vi "CRYUnflatten Results.vi"(11 "Unflatten Result":string) -> (0 "Error?":bool, 2 "Result":T2={"Name"="Test for Signal [L]", "Margin"=nan, "unit"="", "Verdict"=FALSE, "Limit"="", "Max/Min"="", "protected"=FALSE, "Step No."=0, "Test Info"="", "AutoProtect"=FALSE} {"Margin" format="%.2f"}, 3 "Header info":T1={"Data type"="Data            ", "Version"=1, "Dimensions"=0})   [LabVIEW 2013]
uses:
  Typedef Control/CRYResult Cluster.ctl
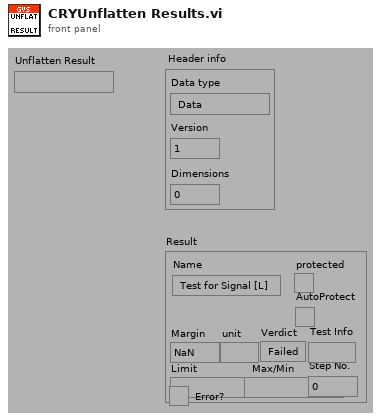
[diagram p1: front panel]
types:
  T1 = cluster{"Data type":string, "Version":u16, "Dimensions":u8}
  T2 = typedef "CRYResult Cluster.ctl" = cluster{"Name":string, "Margin":dbl, "unit":string, "Verdict":bool, "Limit":string, "Max/Min":string, "protected":bool, "Step No.":i32, "Test Info":string, "AutoProtect":bool}
  T3 = cluster{"Name":string, "Margin":dbl, "unit":string, "Verdict":bool, "Limit":string, "Max/Min":string, "protected":bool, "Step No.":i32, "Test Info":string, "AutoProtect":bool}
  T4 = cluster{"unsigned byte array[0]":u8, "unsigned byte array[1]":u8, "unsigned byte array[2]":u8}
  T5 = cluster{"substring":string, u16, "unsigned byte array[2]":u8}
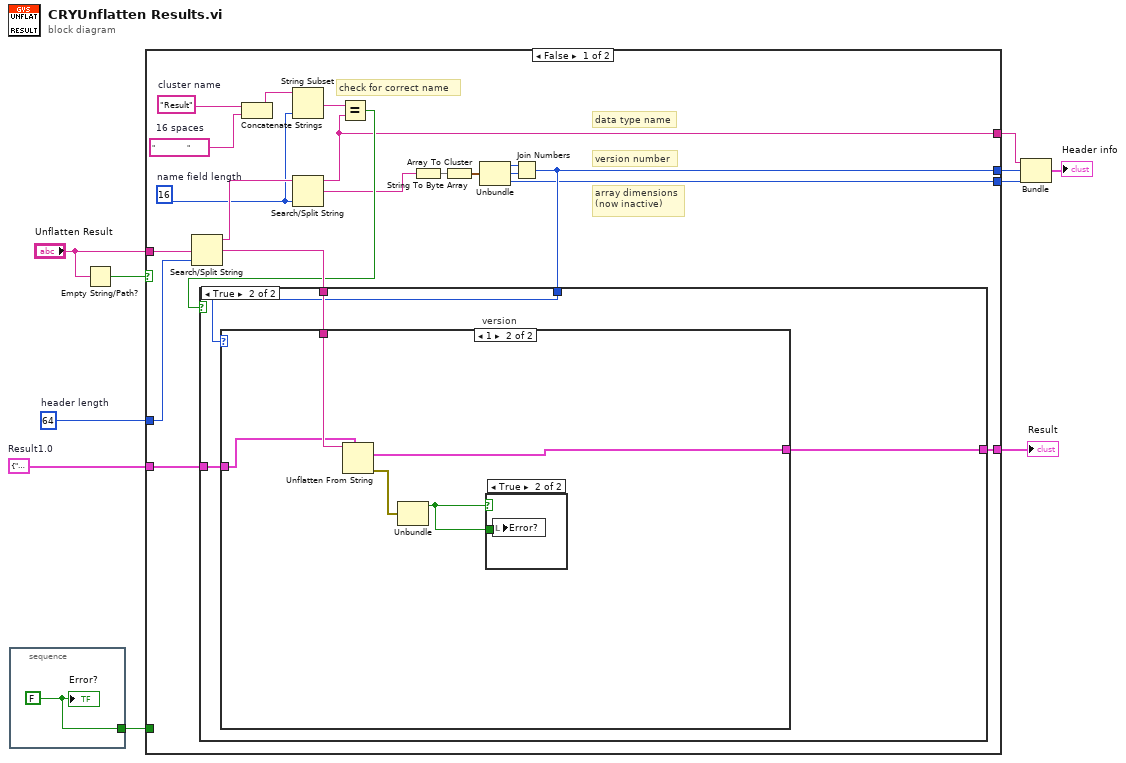
[diagram p0: block diagram]
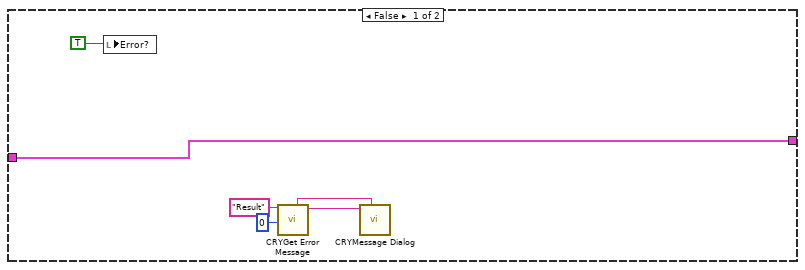
[diagram p2: hidden frame]
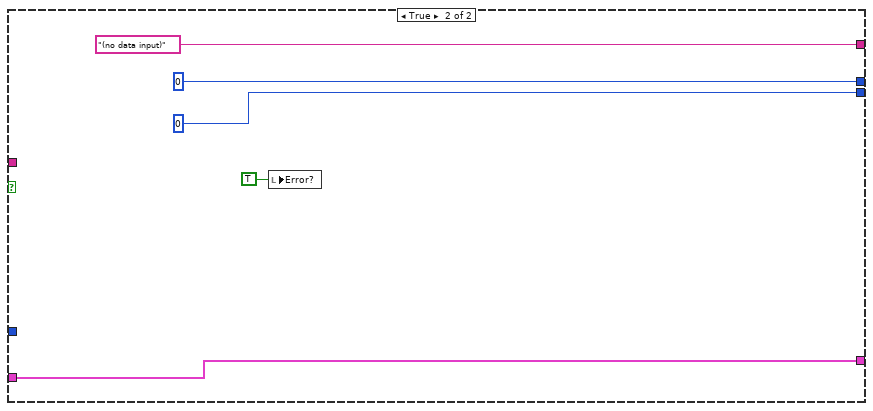
[diagram p5: hidden frame]
diagram:
  w2 = T3 {"Name"="Test for Signal [L]", "Margin"=nan, "unit"="", "Verdict"=FALSE, "Limit"="", "Max/Min"="", "protected"=FALSE, "Step No."=0, "Test Info"="", "AutoProtect"=FALSE}  # Result1.0
  w8 = 64  # header length
  n1 = stacked-sequence {
    tunnel: [w11] -> w3
    frame #0 {
      w11 = FALSE
      "Error?" <- w11
    }
  }
  n2 = Empty String/Path?(string/path="Unflatten Result") -> (empty?=w9:bool)
  n3 = case shown="False" w9 {
    tunnel: "Unflatten Result" -> [w31 _]
    tunnel: w8 -> [w25 _]
    tunnel: [w22 u16 0] -> w6
    tunnel: [w14 u8 0] -> w7
    tunnel: [w15 "(no data input)" ("substring")] -> w5
    tunnel: w3 -> [_ _]
    tunnel: [w13 w49] -> w1
    tunnel: w2 -> [w12 w49]
    frame False {
      w19 = "                "  # 16 spaces
      w20 = "Result"  # cluster name
      w17 = 16  # name field length
      # "check for correct name"
      # "array dimensions\n(now inactive)"
      # "version number"
      # "data type name"
      n4 = Search/Split String(string=w31, offset (0)=w25) -> (substring before match=w24:string, match + rest of string=w26:string)  [unwired: 2 out]
      n5 = Concatenate Strings(w20, w19) -> (w18:string)
      n6 = String Subset(string=w18, length (rest)=w17) -> (substring=w16:string)  [unwired: 1 out]
      n7 = Search/Split String(string=w24, offset (0)=w17) -> (substring before match=w15:string, match + rest of string=w21:string)  [unwired: 2 out]
      n8 = Equal?(x=w16, y=w15) -> (x = y?=w23:bool)
      n9 = String To Byte Array(string=w21) -> (unsigned byte array=w30:u8[])
      n10 = Array To Cluster(array=w30) -> (cluster=w29:T4)
      n11 = Unbundle(w29) -> ("unsigned byte array[0]"=w28:u8, "unsigned byte array[1]"=w27:u8, "unsigned byte array[2]"=w14:u8)
      n12 = Join Numbers(hi=w28, lo=w27) -> ((hi.lo)=w22:u16)
      n13 = case shown="True" w23 {
        tunnel: w26 -> [_ w41]
        tunnel: w22 -> [_ w40]
        tunnel: [w36 w39] -> w13
        tunnel: w12 -> [w36 w38]
        frame False {
          n14 = local write "Error?"(TRUE) -> ()
          n15 = call "CRYGet Error Message.vi"("Error No"=0 ("No"), "Kind"="Result") -> ("Message"=w33:string, "Window Title"=w32:string)  [unwired: 4 in, 4 out]
          n16 = call "CRYMessage Dialog.vi"("Window Title"=w32, "Message Content"=w33) -> ()  [unwired: 8 in, 2 out]
        }
        frame True {
          n17 = case "version" shown="1" w40 {
            tunnel: w41 -> [_ w47]
            tunnel: [w42 w44] -> w39
            tunnel: w38 -> [w42 w45]
            frame Default {
            }
            frame 1 {
              n18 = Unflatten From String(type=w45, binary string=w47) -> (value=w44:T3, error out=w43:errorcluster)  [unwired: 1 in, 3 out]
              n19 = Unbundle(w43) -> ("status"=w46:bool)  [unwired: 2 out]
              n20 = case shown="True" w46 {
                tunnel: w46 -> [_ w48]
                frame False {
                }
                frame True {
                  n21 = local write "Error?"(w48) -> ()
                }
              }
            }
          }
        }
      }
    }
    frame True {
      n22 = local write "Error?"(TRUE ("Error?")) -> ()
    }
  }
  "Result" <- w1
  n23 = Bundle("substring"=w5, w6, "unsigned byte array[2]"=w7) -> (→"Header info":T5)  [unwired: 1 out]
